vi "DQMH_Hardware Selection.vi"(11 "File Path":path) -> (3 "Data out":T5)   [LabVIEW 2025]
uses:
  Libraries/USB IO/Classes/Hardware Selection.ctl
  Libraries/Power Supply/Classes/hardware-selection.ctl
  0247f9e0-db19-4a48-b89f-65ca14ef11bb.vi
  <vilib>/JDP Science/JSONtext/JSON text to Variant.vi
  <vilib>/JDP Science/JSONtext/LVClass Serializer/JSONtext LVClass Serializer.lvclass
  Libraries/Motor/Classes/Stepper/Motor Selection.ctl
  Libraries/Wheatstone Bridge/Wheatstone Bridge/Hardware Selection.ctl
  Libraries/Wheatstone Bridge/Wheatstone Bridge/Wheatstone Bridge.lvclass
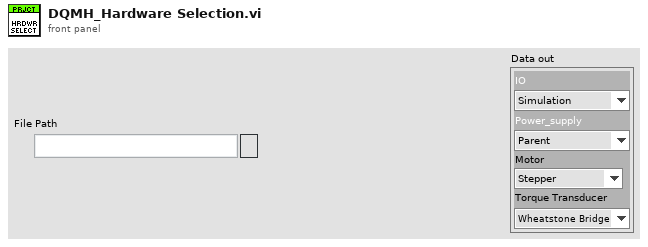
[diagram p1: front panel]
types:
  T1 = typedef "Hardware Selection.ctl" = enum16{"Simulation", "USB-6000", "USB-6001", "Arduino Uno"}
  T2 = typedef "hardware-selection.ctl" = enum16{"Parent", "Simulation", "PSP-603"}
  T3 = typedef "Motor Selection.ctl" = enum16{"Stepper", "CL57RS"}
  T4 = typedef "Wheatstone Bridge.lvlib/Wheatstone Bridge.lvclass/Hardware Selection.ctl" = enum16{"Wheatstone Bridge", "NI-9237"}
  T5 = cluster{"IO":T1, "Power_supply":T2, "Motor":T3, "Torque Transducer":T4}
  T6 = cluster{"IO":T1, "Power_supply":T2, "Motor":T3, "Torque_Transducer":T4}
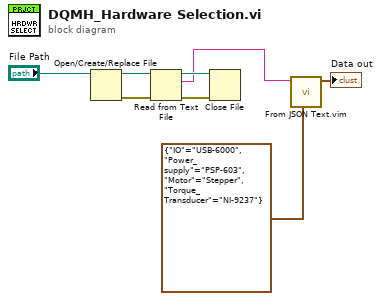
[diagram p0: block diagram]
diagram:
  n1 = Open/Create/Replace File(file path (use dialog)="File Path") -> (refnum out=w6:refnum<file>, error out=w7:errorcluster)  [unwired: 5 in, 1 out]
  n2 = Read from Text File(file (use dialog)=w6, error in=w7) -> (refnum out=w4:refnum<file>, text=w3:string, error out=w5:errorcluster)  [unwired: 2 in, 1 out]
  n3 = Close File(refnum=w4, error in=w5) -> ()  [unwired: 2 out]
  n4 = call "From JSON Text.vim"("Data Type and Default Value"=T6 {"IO"=enum."USB-6000", "Power_supply"=enum."PSP-603", "Motor"=enum."Stepper", "Torque_Transducer"=enum."NI-9237"}, "JSON"=w3) -> ("Data out"=→"Data out":T6)  [unwired: 8 in, 1 out]
